vi "Batch Channel Settings Dialog.vi"(8 "error in (no error)":errorcluster) -> (0 "error out":errorcluster, 1 "Mode selected":T1, 2 "channels selected":i32, 3 "Selected name":string, 4 "Default Value":dbl, 5 "Temp params":T2={"A"=0.003908299840986729, "B"=-5.774999749519338e-07, "C"=-4.182999866625403e-12, "R0"=1000.0}, 7 "Create bank channels":bool)   [LabVIEW 2011, in "NI 272x Resistive Simulation Custom Device Configuration.lvlib"]
uses:
  NI 272x Resistive Simulation Custom Device Configuration.lvlib
  Controls/Device Type.ctl
  Controls/Channel Mode.ctl
  <instrlib>/ni272xReferenceVIs/ni272xReferenceVIs.llb/ni272x Callendar-Van Dusen RTD Parameters.ctl
  NI 272x Resistive Simulation Custom Device Shared.lvlib
panel:
  in  "Device Name":string
  in  "Default Desired Value":dbl
  in  "ConChns":bool=TRUE
  in  "# Channels":i32
  in  "temp param":T2={"A"=0.00139999995008111, "B"=0.00023700000019744039, "C"=9.899999753315569e-08, "R0"=1000.0} caption="Callendar-Van Dusen RTD\n parameters"
  in  "Mode":T1
  in  "Device Type":T3
  in  "OK":bool
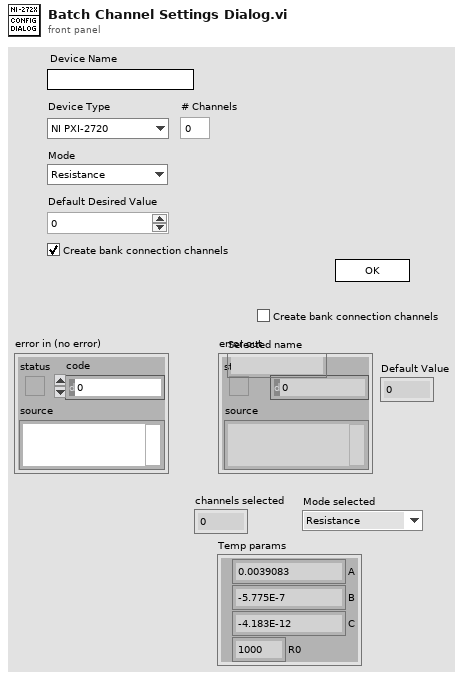
[diagram p1: front panel]
types:
  T1 = typedef "NI 272x Resistive Simulation Custom Device Shared.lvlib/Channel Mode.ctl" = enum16{"Resistance", "RTD Temperature"}
  T2 = typedef "ni272x Callendar-Van Dusen RTD Parameters.ctl" = cluster{"A":dbl, "B":dbl, "C":dbl, "R0":dbl}
  T3 = typedef "NI 272x Resistive Simulation Custom Device Configuration.lvlib/Device Type.ctl" = enum16{"NI PXI-2720", "NI PXI-2722", "NI PXIe-2725", "NI PXIe-2727", "Custom"}
  T4 = enum8{"Enabled", "Disabled", "Disabled and Grayed Out"}
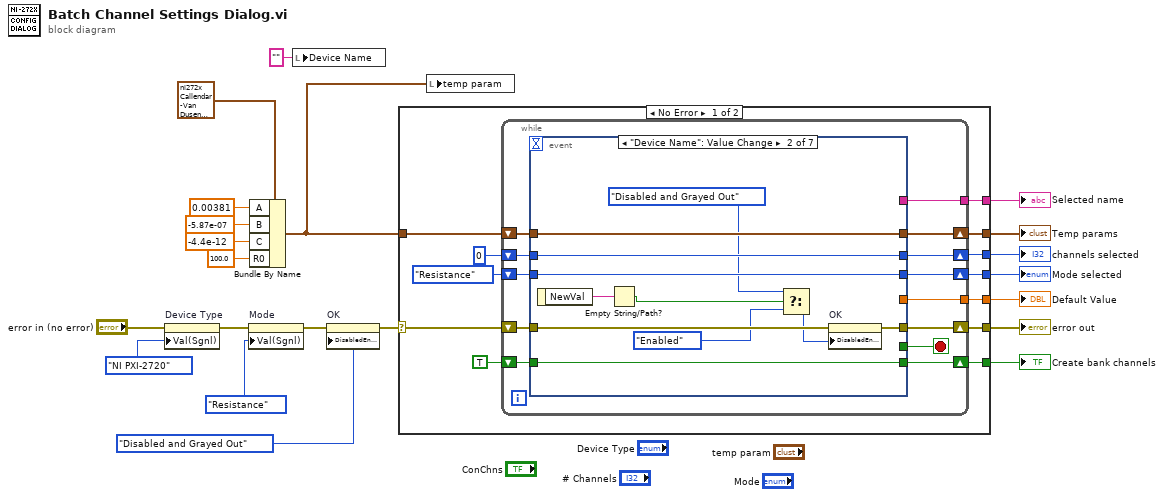
[diagram p0: block diagram]
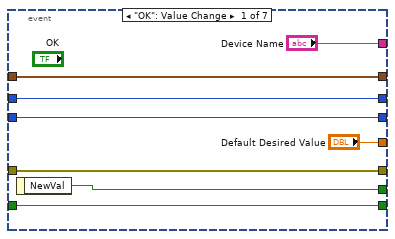
[diagram p2: hidden frame]
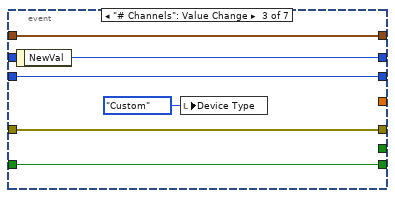
[diagram p3: hidden frame]
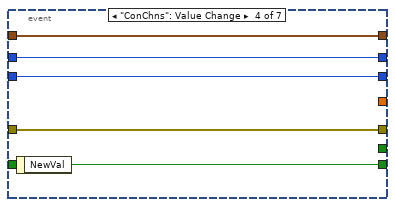
[diagram p4: hidden frame]
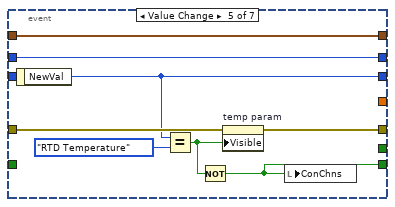
[diagram p5: hidden frame]
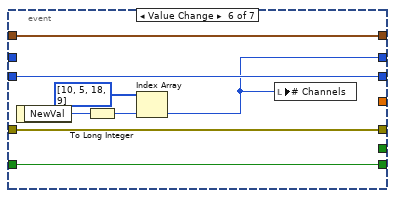
[diagram p6: hidden frame]
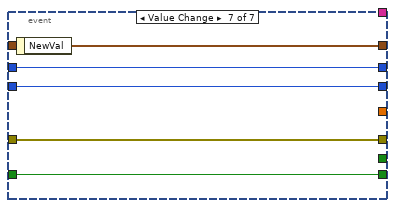
[diagram p7: hidden frame]
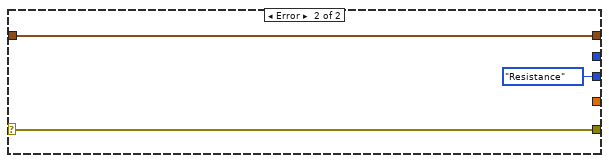
[diagram p8: hidden frame]
diagram:
  n1 = property on="Device Type" class="Enum (strict)"(error in="error in (no error)", "Val(Sgnl)"=Device_Type."NI PXI-2720" ("Value (Signaling)")) -> (error out=w15:errorcluster)  [unwired: 1 in, 1 out]
  n2 = property on="Mode" class="Enum (strict)"(error in=w15, "Val(Sgnl)"=Channel_Mode."Resistance" ("Mode")) -> (error out=w3:errorcluster)  [unwired: 1 in, 1 out]
  n3 = Bundle By Name(cluster=T2 {"A"=0.003908299840986729, "B"=-5.774999749519338e-07, "C"=-4.182999866625403e-12, "R0"=1000.0} ("temp param"), "A"=0.00381, "B"=-5.87e-07, "C"=-4.4e-12, "R0"=100.0) -> (w6:T2)
  n4 = local write "Device Name"("" ("Device Name")) -> ()
  n5 = property on="OK" class="Bool"(error in=w3, "DisabledEnum"=T4."Disabled and Grayed Out" ("Disabled")) -> (error out=w4:errorcluster)  [unwired: 1 in, 1 out]
  n6 = case shown="No Error" w4 {
    selector: w4 -> [w29 w100]
    tunnel: w6 -> [w33 w99]
    tunnel: [w32 w100] -> w20
    tunnel: [w31 w99] -> w19
    tunnel: [w30 _] -> w18
    tunnel: [w26 Channel_Mode."Resistance" ("Mode")] -> w17
    tunnel: [w24 _] -> w16
    tunnel: [w23 _] -> w7
    tunnel: [w22 _] -> w5
    frame No Error {
      n7 = while {
        shift-right: [w45] -> w31
        shift-left: w33 -> [w44]
        shift-right: [w43] -> w30
        shift-left: 0 ("# Channels") -> [w42]
        shift-right: [w40] -> w32
        shift-left: w29 -> [w41]
        shift-right: [w39] -> w26
        shift-left: Channel_Mode."Resistance" ("Mode") -> [w38]
        shift-right: [w37] -> w24
        shift-left: TRUE -> [w36]
        tunnel: [w35] -> w23
        tunnel: [w34] -> w22
        stop <- w46 stop-if-true
        n8 = event shown="[1] \"Device Name\": Value Change" {
          selector: _ -> [_ _ _ _ _ _ _]
          dyn-events: _ -> [_ _ _ _ _ _ _]
          timeout: _ -> [_ _ _ _ _ _ _]
          tunnel: [w50 _ _ _ _ _ _] -> w46
          tunnel: [w54 w65 w71 w76 w84 w92 w94] -> w45
          tunnel: w44 -> [w54 w65 w71 w76 w84 w92 _]
          tunnel: [w53 w64 w70 w75 w83 w88 w97] -> w43
          tunnel: w42 -> [w53 w64 _ w75 w83 _ w97]
          tunnel: w41 -> [w52 w59 w69 w74 w82 w90 w96]
          tunnel: [w52 w60 w69 w74 w79 w90 w96] -> w40
          tunnel: [w51 w63 w68 w73 w80 w89 w95] -> w39
          tunnel: w38 -> [w51 w63 w68 w73 _ w89 w95]
          tunnel: [w49 w62 w67 w72 w77 w86 w93] -> w37
          tunnel: w36 -> [w49 w62 w67 _ _ w86 w93]
          tunnel: ["Default Desired Value" _ _ _ _ _ _] -> w35
          tunnel: ["Device Name" _ _ _ _ _ _] -> w34
          event "OK": Value Change {
            n9 = event-data() -> ("NewVal"=w50:bool)  [unwired: 1 in]
          }
          event "Device Name": Value Change {
            n10 = event-data() -> ("NewVal"=w61:string)  [unwired: 1 in]
            n11 = Empty String/Path?(string/path=w61) -> (empty?=w58:bool)
            n12 = Select(t=T4."Disabled and Grayed Out", s=w58, f=T4."Enabled" ("Disabled")) -> (s? t:f=w55:T4)
            n13 = property on="OK" class="Bool"(error in=w59, "DisabledEnum"=w55) -> (error out=w60:errorcluster)  [unwired: 1 in, 1 out]
          }
          event "# Channels": Value Change {
            n14 = event-data() -> ("NewVal"=w70:i32)  [unwired: 1 in]
            n15 = local write "Device Type"(Device_Type."Custom" ("Device Type")) -> ()
          }
          event "ConChns": Value Change {
            n16 = event-data() -> ("NewVal"=w72:bool)  [unwired: 1 in]
          }
          event Value Change {
            n17 = event-data() -> ("NewVal"=w80:T1)  [unwired: 1 in]
            n18 = Equal?(x=w80, y=Channel_Mode."RTD Temperature" ("Mode")) -> (x = y?=w78:bool)
            n19 = Not(x=w78) -> (.not. x?=w77:bool)
            n20 = property on="temp param" class="Clust (strict)"(error in=w82, "Visible"=w78) -> (error out=w79:errorcluster)  [unwired: 1 in, 1 out]
            n21 = local write "ConChns"(w77) -> ()
          }
          event Value Change {
            n22 = event-data() -> ("NewVal"=w87:T3)  [unwired: 1 in]
            n23 = To Long Integer(number=w87) -> (32bit integer=w91:i32)
            n24 = Index Array(array=i32[] [10, 5, 18, 9] ("Device Information"), index=w91) -> (element=w88:i32)
            n25 = local write "# Channels"(w88) -> ()
          }
          event Value Change {
            n26 = event-data() -> ("NewVal"=w94:T2)  [unwired: 1 in]
          }
        }
      }
    }
    frame Error {
    }
  }
  "error out" <- w20
  "Temp params" <- w19
  "channels selected" <- w18
  "Mode selected" <- w17
  "Create bank channels" <- w16
  "Default Value" <- w7
  "Selected name" <- w5
  n27 = local write "temp param"(w6) -> ()
